vi "LabView_abd_IoT.vi"() -> ()   [LabVIEW 2015]
panel:
  in  "stop":bool
  out "Link Quality":sgl
  out "Battery Voltage":sgl
  out "AI0":sgl
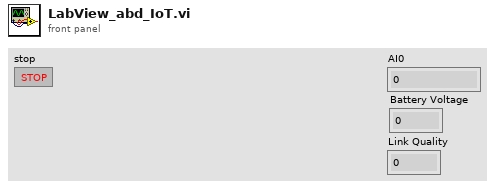
[diagram p1: front panel]
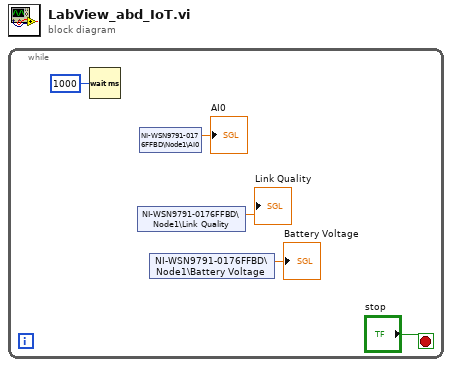
[diagram p0: block diagram]
diagram:
  n1 = while {
    stop <- "stop" stop-if-true
    n2 = Wait (ms)(milliseconds to wait=u32 1000) -> ()  [unwired: 1 out]
    n3 = shared-variable "NI-WSN9791-0176FFBD\\Node1\\Link Quality"() -> (→"Link Quality":sgl)  [unwired: 1 in, 1 out]
    n4 = shared-variable "NI-WSN9791-0176FFBD\\Node1\\AI0"() -> (→"AI0":sgl)  [unwired: 1 in, 1 out]
    n5 = shared-variable "NI-WSN9791-0176FFBD\\Node1\\Battery Voltage"() -> (→"Battery Voltage":sgl)  [unwired: 1 in, 1 out]
  }
